vi "Vacuum Test - Step 5.vi"(7 "Step":i32, 8 "error in":errorcluster, 9 "Test Results In":T9, 10 "PAS In":T8 caption="Gas", 11 "Test Configuration":T1) -> (0 "error out":errorcluster, 1 "Test Results Out":T9, 2 "PAS Out":T8 caption="Gas", 3 "Test Configuration Out":T1)   [LabVIEW 2015]
uses:
  CAN Communication/PAS/Typedefs/Session Handle.ctl
  CAN Communication/PAS/PAS.lvclass
  Controls/Test Results.ctl
  Controls/Step Result.ctl
  Controls/Test Configuration.ctl
  Controls/Vacuum Test.ctl
  Controls/Test Timing.ctl
  Controls/Vaccum Thresholds.ctl
  Controls/Helium Test.ctl
  Controls/Helium Thresholds.ctl
  Controls/Functional Test.ctl
  CAN Communication/PAS/Typedefs/Valves.ctl
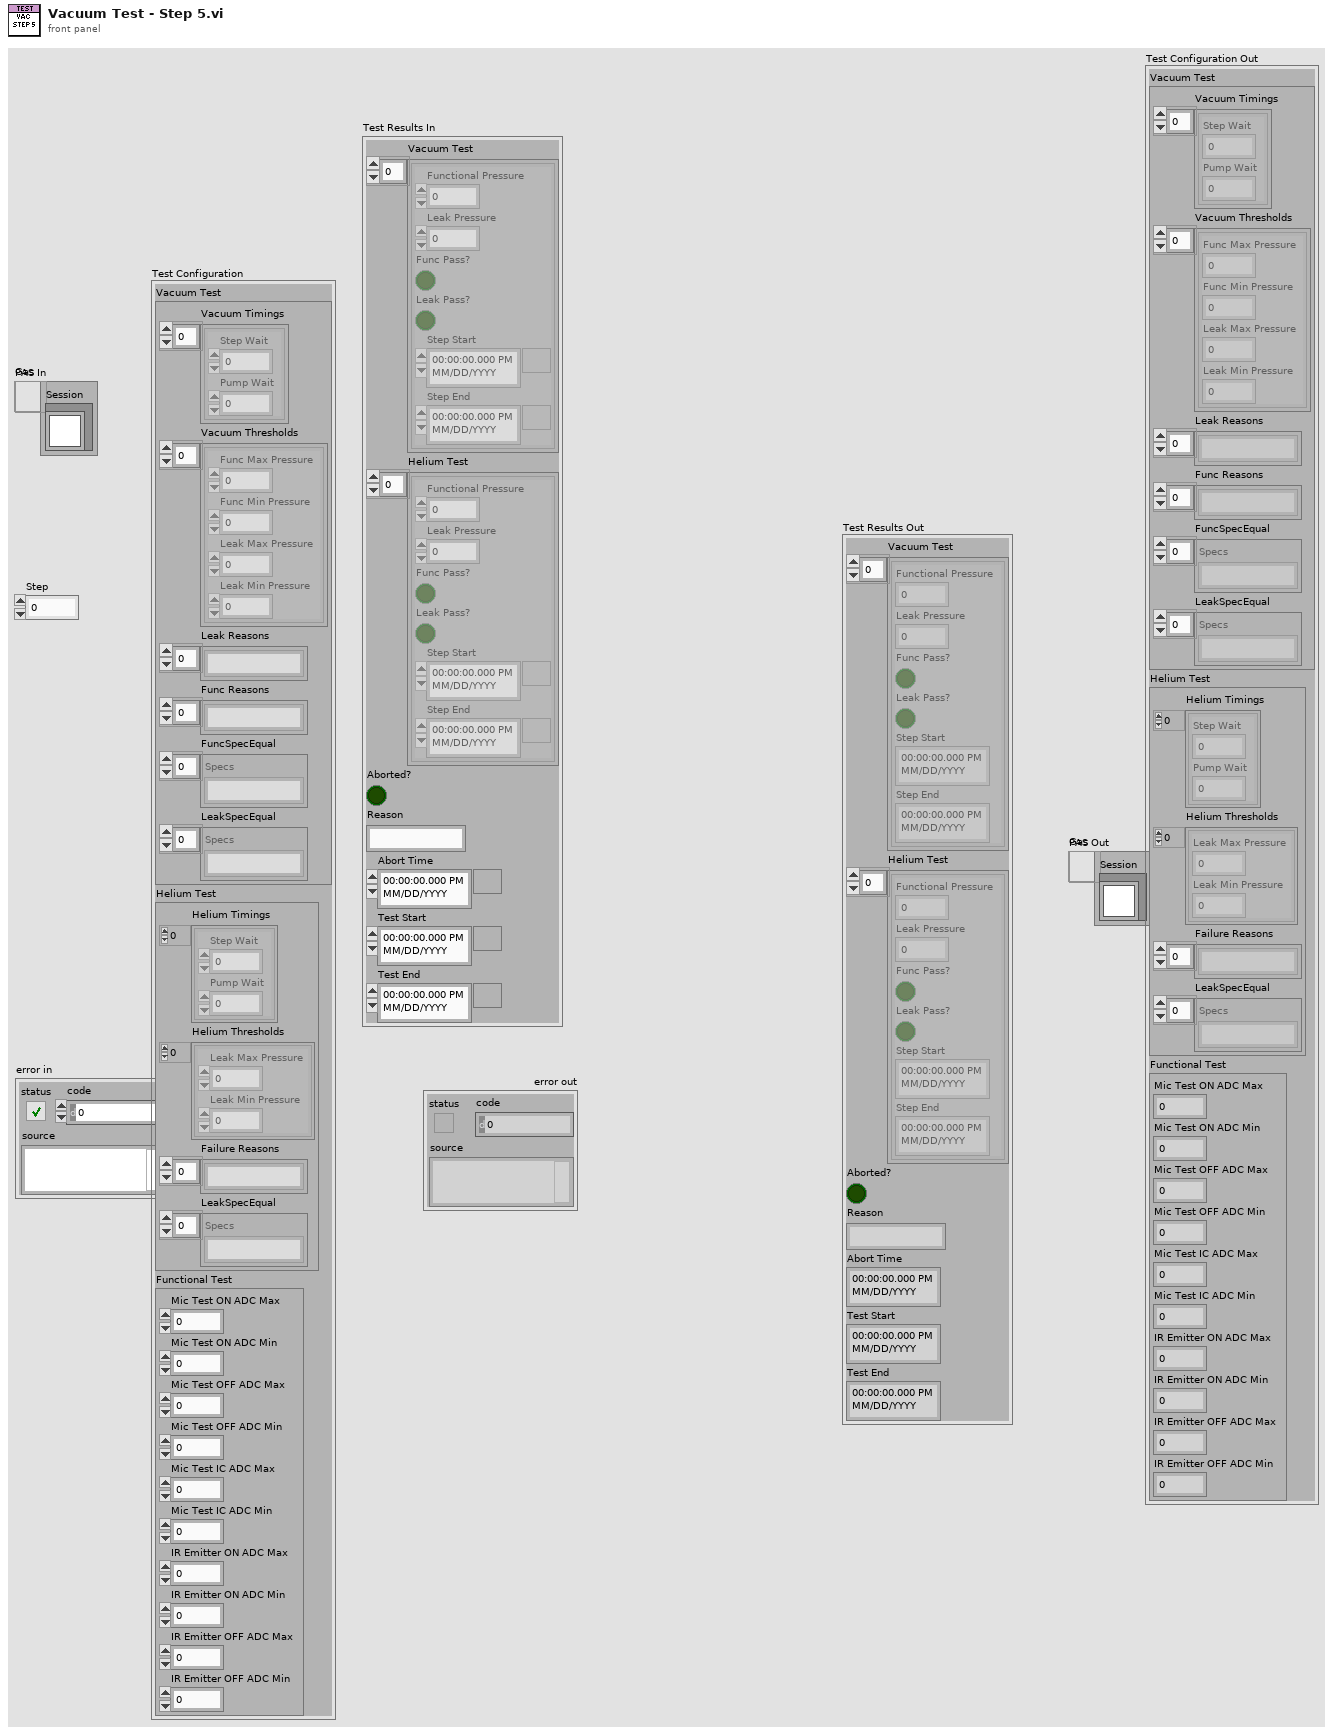
[diagram p1: front panel]
types:
  T1 = typedef "Test Configuration.ctl" = cluster{"Vacuum Test":T2, "Helium Test":T5, "Functional Test":T7}
  T2 = typedef "Vacuum Test.ctl" = cluster{"Vacuum Timings":T3[], "Vacuum Thresholds":T4[], "Leak Reasons":string[], "Func Reasons":string[], "FuncSpecEqual":string[], "LeakSpecEqual":string[]}
  T3 = typedef "Test Timing.ctl" = cluster{"Step Wait":dbl, "Pump Wait":dbl}
  T4 = typedef "Vaccum Thresholds.ctl" = cluster{"Func Max Pressure":dbl, "Func Min Pressure":dbl, "Leak Max Pressure":dbl, "Leak Min Pressure":dbl}
  T5 = typedef "Helium Test.ctl" = cluster{"Helium Timings":T3[], "Helium Thresholds":T6[], "Failure Reasons":string[], "LeakSpecEqual":string[]}
  T6 = typedef "Helium Thresholds.ctl" = cluster{"Leak Max Pressure":dbl, "Leak Min Pressure":dbl}
  T7 = typedef "Functional Test.ctl" = cluster{"Mic Test ON ADC Max":dbl, "Mic Test ON ADC Min":dbl, "Mic Test OFF ADC Max":dbl, "Mic Test OFF ADC Min":dbl, "Mic Test IC ADC Max":dbl, "Mic Test IC ADC Min":dbl, "IR Emitter ON ADC Max":dbl, "IR Emitter ON ADC Min":dbl, "IR Emitter OFF ADC Max":dbl, "IR Emitter OFF ADC Min":dbl}
  T8 = typedef "PAS.lvclass/Session Handle.ctl" = refnum<data-value>
  T9 = typedef "Test Results.ctl" = cluster{"Vacuum Test":T10[], "Helium Test":T10[], "Aborted?":bool, "Reason":string, "Abort Time":timestamp, "Test Start":timestamp, "Test End":timestamp}
  T10 = typedef "Step Result.ctl" = cluster{"Functional Pressure":dbl, "Leak Pressure":dbl, "Func Pass?":bool, "Leak Pass?":bool, "Step Start":timestamp, "Step End":timestamp}
  T11 = typedef "PAS.lvclass/Valves.ctl" = u16
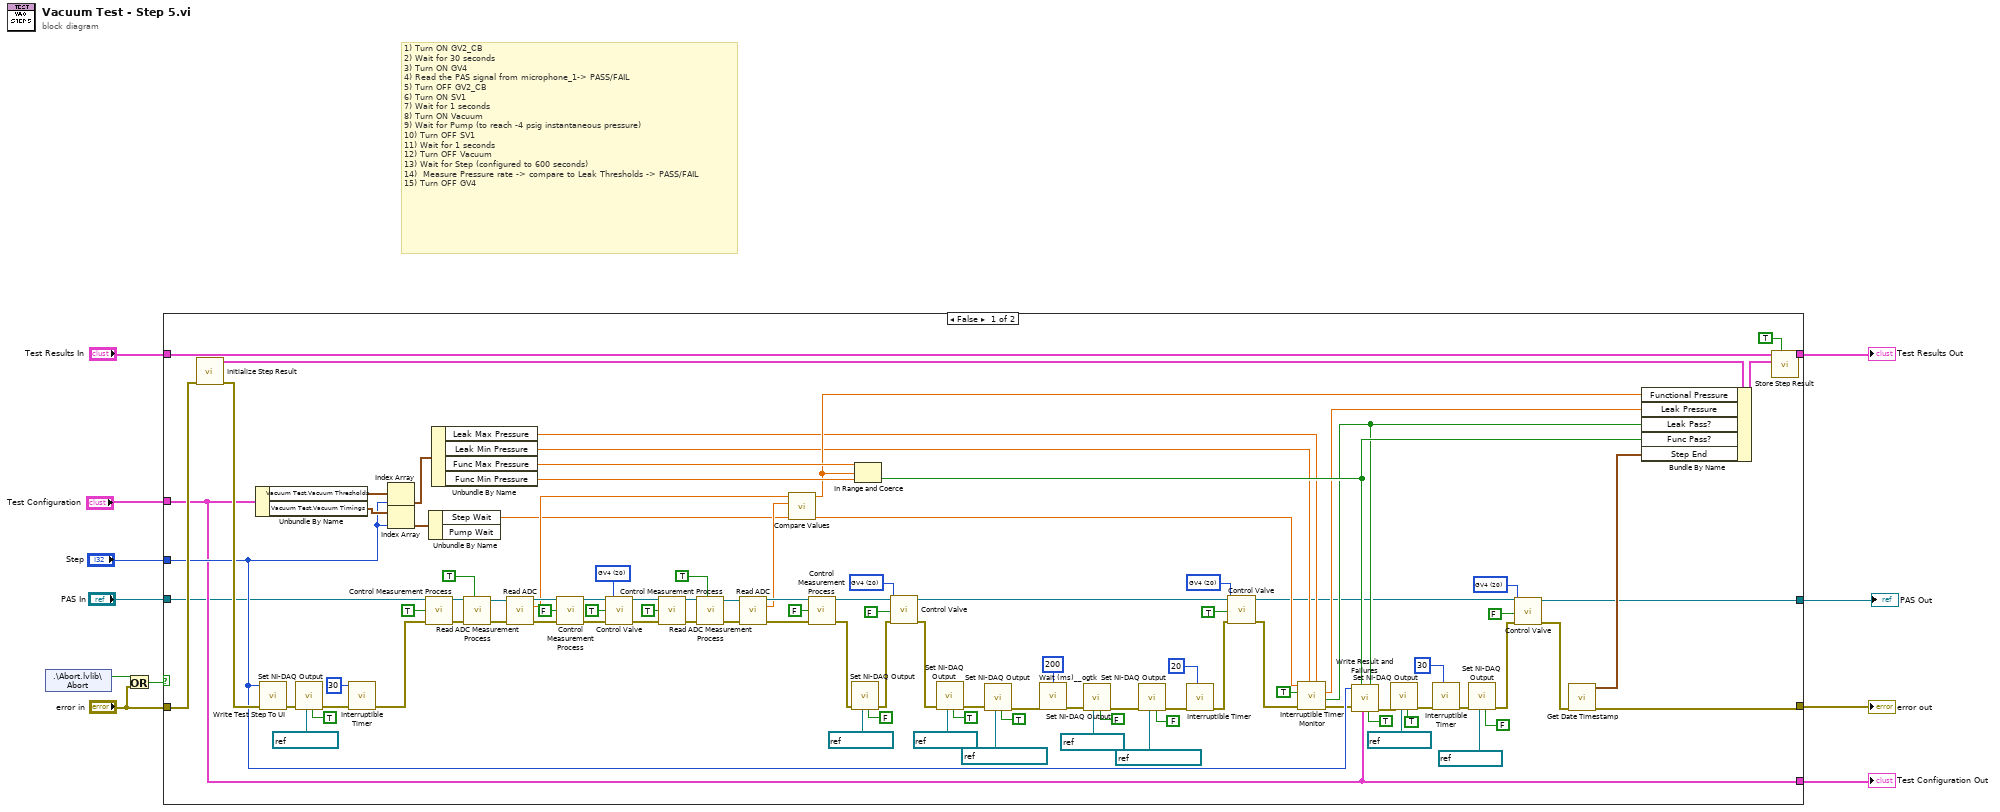
[diagram p0: block diagram]
diagram:
  # "1) Turn ON GV2_CB\n2) Wait for 30 seconds\n3) Turn ON GV4\n4) Read the PAS signal from microphone_1-> PASS/FAIL\n5) Turn OFF GV2_CB\n6) Turn ON SV1\n7) Wait for 1 seconds\n8) Turn ON Vacuum\n9) Wait for Pump (to reach -4 psig instantaneous pressure)\n10) Turn OFF SV1\n11) Wait for 1 seconds\n12) Turn OFF Vacuum\n13) Wait for Step (configured to 600 seconds)\n14)  Measure Pressure rate -> compare to Leak Thresholds -> PASS/FAIL\n15) Turn OFF GV4"
  n1 = shared-variable ".\\Abort.lvlib\\Abort"() -> (w10:bool)  [unwired: 1 in, 1 out]
  n2 = Or(x=w10, y="error in") -> (x .or. y?=w9:bool)
  n3 = case shown="False" w9 {
    tunnel: "error in" -> [w113 w116]
    tunnel: "Test Results In" -> [w110 w117]
    tunnel: [w111 w117] -> w7
    tunnel: [w13 w116] -> w6
    tunnel: "Test Configuration" -> [w91 w115]
    tunnel: "Step" -> [w101 _]
    tunnel: [w91 w115] -> w1
    tunnel: [w82 w114] -> w3
    tunnel: "PAS In" -> [w66 w114]
    frame False {
      w20 = T11 20 items=["GV1"=17, "GV2"=18, "GV3"=19, "GV4"=20] ("Valves")
      w28 = T11 20 items=["GV1"=17, "GV2"=18, "GV3"=19, "GV4"=20] ("Valves")
      w74 = T11 20 items=["GV1"=17, "GV2"=18, "GV3"=19, "GV4"=20] ("Valves")
      w84 = T11 20 items=["GV1"=17, "GV2"=18, "GV3"=19, "GV4"=20] ("Valves")
      n4 = call "Initialize Step Result.vi"("error in (no error)"=w113) -> ("error out"=w112:errorcluster, "New Step Result"=w109:T10)  [unwired: 8 in, 1 out]
      n5 = Unbundle By Name(w91) -> ("Vacuum Test.Vacuum Thresholds"=w106:T4[], "Vacuum Test.Vacuum Timings"=w105:T3[])
      n6 = call "Write Test Step To UI.vi"("error in (no error)"=w112, "Step"=w101) -> ("error out"=w99:errorcluster)  [unwired: 9 in]
      n7 = call "Set NI-DAQ Output.vi"("State"=TRUE, "Channel"=refnum<k21> "GV2_PAS", "error in (no error)"=w99) -> ("error out"=w98:errorcluster)  [unwired: 8 in]
      n8 = call "Interruptible Timer.vi"("error in (no error)"=w98, "Wait (s)"=30) -> ("error out"=w65:errorcluster)  [unwired: 7 in, 2 out]
      n9 = Index Array(array=w106, index=w101) -> (element=w102:T4)
      n10 = Index Array(array=w105, index=w101) -> (element=w104:T3)
      n11 = call "Control Measurement Process.vi"("Session Handle in"=w66, "Start?"=TRUE, "error in (no error)"=w65) -> ("Session Handle out"=w57:T8, "error out"=w56:errorcluster)  [unwired: 9 in, 2 out]
      n12 = Unbundle By Name(w104) -> ("Step Wait"=w34:dbl)  [unwired: 1 out]
      n13 = Unbundle By Name(w102) -> ("Leak Max Pressure"=w32:dbl, "Leak Min Pressure"=w33:dbl, "Func Max Pressure"=w63:dbl, "Func Min Pressure"=w62:dbl)
      n14 = call "Read ADC Measurement Process.vi"("Measurement Started?"=TRUE, "error in (no error)"=w56, "Session Handle in"=w57) -> ("error out"=w54:errorcluster, "Session Handle out"=w55:T8)  [unwired: 6 in, 1 out]
      n15 = call "Read ADC.vi"("Session Handle in"=w55, "error in (no error)"=w54) -> ("Session Handle out"=w79:T8, "ADC"=w61:dbl, "error out"=w78:errorcluster)  [unwired: 10 in, 1 out]
      n16 = call "Control Measurement Process.vi"("Session Handle in"=w79, "Start?"=FALSE, "error in (no error)"=w78) -> ("Session Handle out"=w76:T8, "error out"=w75:errorcluster)  [unwired: 9 in, 2 out]
      n17 = call "Control Valve.vi"("Session Handle in"=w76, "Valves"=w74, "Energize?"=TRUE, "error in (no error)"=w75) -> ("Session Handle out"=w71:T8, "error out"=w70:errorcluster)  [unwired: 8 in, 2 out]
      n18 = call "Control Measurement Process.vi"("Session Handle in"=w71, "Start?"=TRUE, "error in (no error)"=w70) -> ("Session Handle out"=w52:T8, "error out"=w50:errorcluster)  [unwired: 9 in, 2 out]
      n19 = call "Read ADC Measurement Process.vi"("Measurement Started?"=TRUE, "error in (no error)"=w50, "Session Handle in"=w52) -> ("error out"=w49:errorcluster, "Session Handle out"=w51:T8)  [unwired: 6 in, 1 out]
      n20 = call "Read ADC.vi"("Session Handle in"=w51, "error in (no error)"=w49) -> ("Session Handle out"=w69:T8, "ADC"=w60:dbl, "error out"=w68:errorcluster)  [unwired: 10 in, 1 out]
      n21 = call "Compare Values.vi"("P2"=w60, "P1"=w61) -> ("Abs Diff"=w58:dbl)  [unwired: 9 in]
      n22 = call "Control Measurement Process.vi"("Session Handle in"=w69, "Start?"=FALSE, "error in (no error)"=w68) -> ("Session Handle out"=w26:T8, "error out"=w64:errorcluster)  [unwired: 9 in, 2 out]
      n23 = call "Set NI-DAQ Output.vi"("State"=FALSE, "Channel"=refnum<k21> "GV2_PAS", "error in (no error)"=w64) -> ("error out"=w25:errorcluster)  [unwired: 8 in]
      n24 = In Range and Coerce(upper limit=w63, x=w58, lower limit=w62) -> (In Range?=w59:bool)  [unwired: 1 out]
      n25 = call "Control Valve.vi"("Session Handle in"=w26, "Valves"=w28, "Energize?"=FALSE, "error in (no error)"=w25) -> ("Session Handle out"=w19:T8, "error out"=w24:errorcluster)  [unwired: 8 in, 2 out]
      n26 = call "Set NI-DAQ Output.vi"("State"=TRUE, "Channel"=refnum<k21> "SV1_PAS", "error in (no error)"=w24) -> ("error out"=w47:errorcluster)  [unwired: 8 in]
      n27 = call "Set NI-DAQ Output.vi"("State"=TRUE, "Channel"=refnum<k21> "Vacuum_PAS", "error in (no error)"=w47) -> ("error out"=w46:errorcluster)  [unwired: 8 in]
      n28 = call <userlib>:"Wait (ms)__ogtk.vi"("error in (no error)"=w46, "milliseconds to wait"=u32 200) -> ("error out"=w45:errorcluster)  [unwired: 8 in, 1 out]
      n29 = call "Set NI-DAQ Output.vi"("State"=FALSE, "Channel"=refnum<k21> "SV1_PAS", "error in (no error)"=w45) -> ("error out"=w43:errorcluster)  [unwired: 8 in]
      n30 = call "Set NI-DAQ Output.vi"("State"=FALSE, "Channel"=refnum<k21> "Vacuum_PAS", "error in (no error)"=w43) -> ("error out"=w23:errorcluster)  [unwired: 8 in]
      n31 = call "Interruptible Timer.vi"("error in (no error)"=w23, "Wait (s)"=20) -> ("error out"=w18:errorcluster)  [unwired: 7 in, 2 out]
      n32 = call "Control Valve.vi"("Session Handle in"=w19, "Valves"=w20, "Energize?"=TRUE, "error in (no error)"=w18) -> ("Session Handle out"=w16:T8, "error out"=w17:errorcluster)  [unwired: 8 in, 2 out]
      n33 = call "Interruptible Timer Monitor.vi"("Max"=w32, "Min"=w33, "error in (no error)"=w17, "Update UI?"=TRUE, "Wait (s)"=w34) -> ("error out"=w15:errorcluster, "In Range?"=w29:bool, "Leak Rate"=w31:dbl)  [unwired: 3 in, 1 out]
      n34 = call "Write Result and Failures.vi"("Vacuum?"=TRUE, "Leak"=w29, "Test Configuration"=w91, "Func"=w59, "error in (no error)"=w15, "Step"=w101) -> ("error out"=w14:errorcluster)  [unwired: 5 in]
      n35 = call "Set NI-DAQ Output.vi"("State"=TRUE, "Channel"=refnum<k21> "SV1_PAS", "error in (no error)"=w14) -> ("error out"=w39:errorcluster)  [unwired: 8 in]
      n36 = call "Interruptible Timer.vi"("error in (no error)"=w39, "Wait (s)"=30) -> ("error out"=w37:errorcluster)  [unwired: 7 in, 2 out]
      n37 = call "Set NI-DAQ Output.vi"("State"=FALSE, "Channel"=refnum<k21> "SV1_PAS", "error in (no error)"=w37) -> ("error out"=w30:errorcluster)  [unwired: 8 in]
      n38 = call "Control Valve.vi"("Session Handle in"=w16, "Valves"=w84, "Energize?"=FALSE, "error in (no error)"=w30) -> ("Session Handle out"=w82:T8, "error out"=w81:errorcluster)  [unwired: 8 in, 2 out]
      n39 = call "Get Date Timestamp.vi"("error in (no error)"=w81) -> ("error out"=w13:errorcluster, "current time"=w107:timestamp)  [unwired: 9 in]
      n40 = Bundle By Name(cluster=w109, "Functional Pressure"=w58, "Leak Pressure"=w31, "Leak Pass?"=w29, "Func Pass?"=w59, "Step End"=w107) -> (w108:T10)
      n41 = call "Store Step Result.vi"("Vacuum?"=TRUE, "Step Result"=w108, "Test Results In"=w110) -> ("Test Results Out"=w111:T9)  [unwired: 8 in]
    }
    frame True {
    }
  }
  "error out" <- w6
  "Test Results Out" <- w7
  "PAS Out" <- w3
  "Test Configuration Out" <- w1
